vi "onPrepareJobExecution.vi"(8 "error in (no error)":errorcluster, 11 "Job in":refnum<class "Job.lvclass">) -> (0 "error out":errorcluster, 1 "execution cancelled":bool, 3 "Job out":refnum<class "Job.lvclass">)   [LabVIEW 2013, in "openCronJob.lvlib" / "Job.lvclass"]
uses:
  Job.lvclass
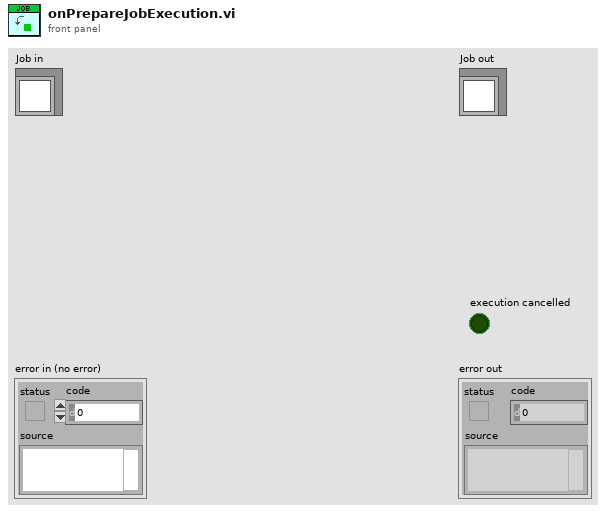
[diagram p1: front panel]
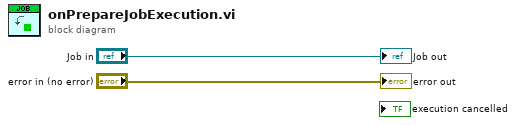
[diagram p0: block diagram]
diagram:
  "error out" <- "error in (no error)"
  "Job out" <- "Job in"
